vi "Bookmark Info Change.vi"(8 "Error In":errorcluster, 11 "Messages In":refnum<queue>) -> (0 "Error Out":errorcluster, 3 "Messages Out":refnum<queue>)   [LabVIEW 2018, in "Bookmark Manager.lvlib"]
uses:
  Bookmark Manager.lvlib
  Controls/Message.ctl
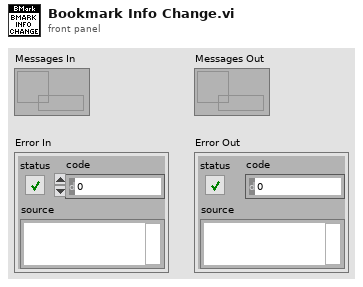
[diagram p1: front panel]
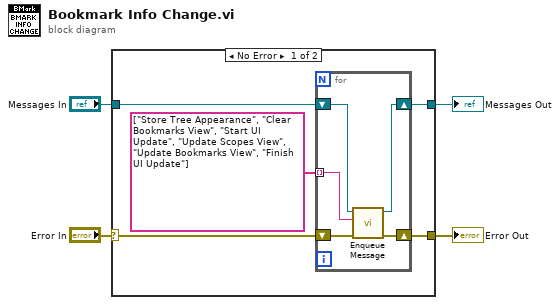
[diagram p0: block diagram]
diagram:
  n1 = case shown="No Error" "Error In" {
    selector: "Error In" -> [w6 w15]
    tunnel: [w5 w15] -> w4
    tunnel: "Messages In" -> [w8 w16]
    tunnel: [w7 w16] -> w2
    frame No Error {
      n2 = for {
        tunnel: string[] ["Store Tree Appearance", "Clear Bookmarks View", "Start UI Update", "Update Scopes View", "Update Bookmarks View", "Finish UI Update"] -> [w14] mode=indexing
        shift-right: [w11] -> w7
        shift-left: w8 -> [w12]
        shift-right: [w13] -> w5
        shift-left: w6 -> [w10]
        n3 = call "Enqueue Message.vi"("Error In"=w10, "Command"=w14, "Message Queue In"=w12) -> ("Error Out"=w13:errorcluster, "Message Queue Out"=w11:refnum<queue>)  [unwired: 7 in]
      }
    }
    frame Error {
    }
  }
  "Error Out" <- w4
  "Messages Out" <- w2
